vi "Day 2.vi"() -> ()   [LabVIEW 2020]
panel:
  out "Array":bool[](array[boolean])
  out "Part 2 sum":i16
  out "Part 1 sum":i16
  out "text":string[](array[string])
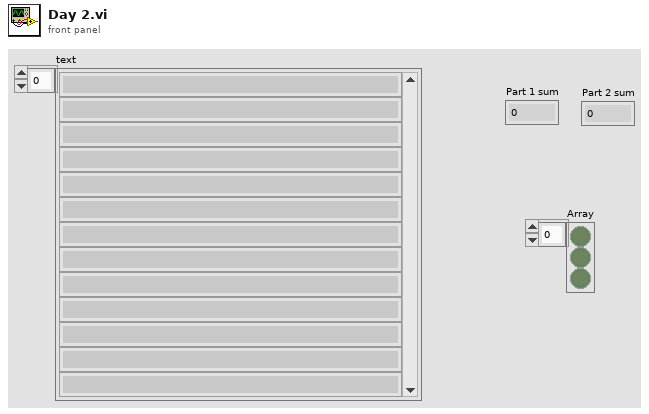
[diagram p1: front panel]
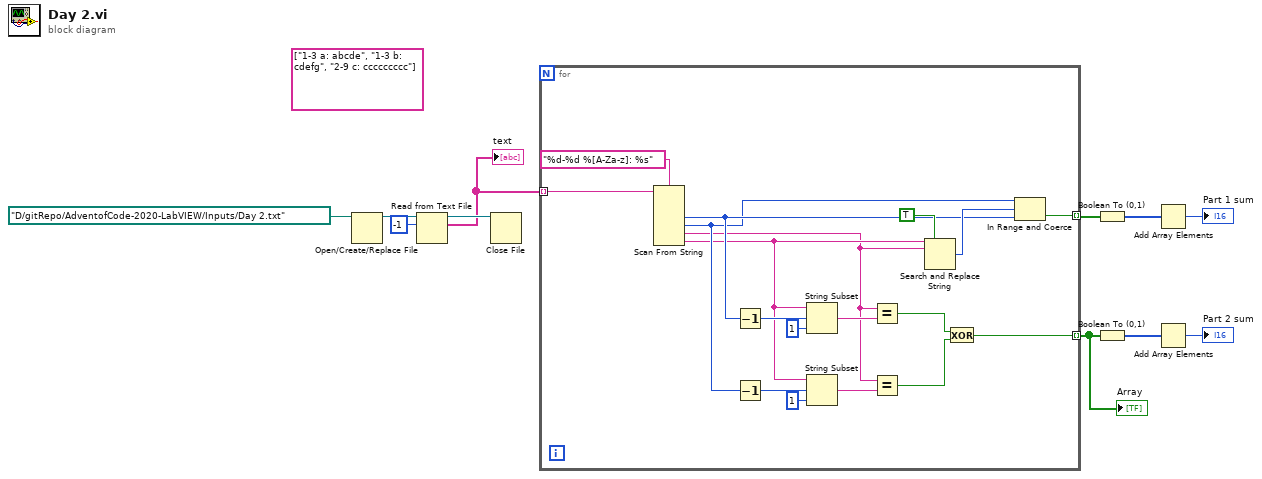
[diagram p0: block diagram]
diagram:
  (unwired) string[] ["1-3 a: abcde", "1-3 b: cdefg", "2-9 c: ccccccccc"] ("text")
  n1 = Open/Create/Replace File(file path (use dialog)=path "D:/gitRepo/AdventofCode-2020-LabVIEW/Inputs/Day 2.txt" ("Path")) -> (refnum out=w10:refnum<file>)  [unwired: 5 in, 2 out]
  n2 = Read from Text File(file (use dialog)=w10, count=-1) -> (refnum out=w9:refnum<file>, text=w1:string[])  [unwired: 2 in, 2 out]
  "text" <- w1
  n3 = Close File(refnum=w9) -> ()  [unwired: 1 in, 2 out]
  n4 = for {
    tunnel: w1 -> [w29] mode=indexing
    tunnel: [w25] -> w7 mode=indexing
    tunnel: [w12] -> w2 mode=indexing
    n5 = Scan From String(format string="%d-%d %[A-Za-z]: %s", input string=w29) -> (output 1=w24:i32, output 2=w19:i32, output 3=w15:string, output 4=w18:string)  [unwired: 6 in, 3 out]
    n6 = Decrement(x=w24) -> (x-1=w23:i32)
    n7 = Decrement(x=w19) -> (x-1=w20:i32)
    n8 = String Subset(string=w18, offset (0)=w23, length (rest)=1 ("length (rest)")) -> (substring=w17:string)
    n9 = String Subset(string=w18, offset (0)=w20, length (rest)=1 ("length (rest)")) -> (substring=w16:string)
    n10 = Equal?(x=w15, y=w17) -> (x = y?=w14:bool)
    n11 = Equal?(x=w15, y=w16) -> (x = y?=w13:bool)
    n12 = Search and Replace String(replace all?=TRUE ("replace all? (F)"), input string=w18, search string=w15) -> (number of replacements=w26:i32)  [unwired: 5 in, 3 out]
    n13 = Exclusive Or(1:w13, 2:w14) -> (0:w12:bool)
    n14 = In Range and Coerce(upper limit=w19, x=w26, lower limit=w24) -> (In Range?=w25:bool)  [unwired: 1 out]
  }
  "Array" <- w2
  n15 = Boolean To (0,1)(Boolean=w7) -> (0, 1=w6:i16[])
  n16 = Boolean To (0,1)(Boolean=w2) -> (0, 1=w3:i16[])
  n17 = Add Array Elements(numeric array=w6) -> (sum=→"Part 1 sum":i16)
  n18 = Add Array Elements(numeric array=w3) -> (sum=→"Part 2 sum":i16)
